vi "Find Axis Instant Velocity.vi"(6 "Sample Period":dbl, 8 "Error In":errorcluster, 10 "Desired Position":dbl, 11 "Current Position":dbl) -> (0 "Error Out":errorcluster, 2 "Axis Velocity":dbl, 3 "Current Position out":dbl)   [LabVIEW 2013]
doc: "This sub-VI determines the instantaneous velocity to send to the motors based on the axis position read\nby the encoders and the position commanded by the system."
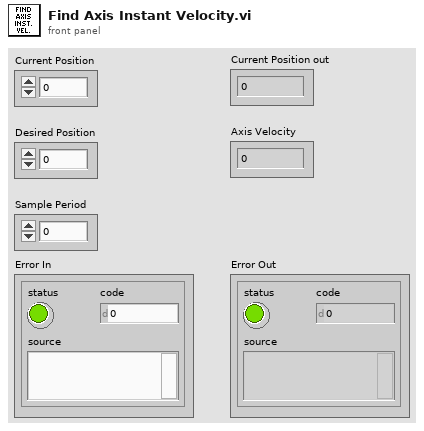
[diagram p1: front panel]
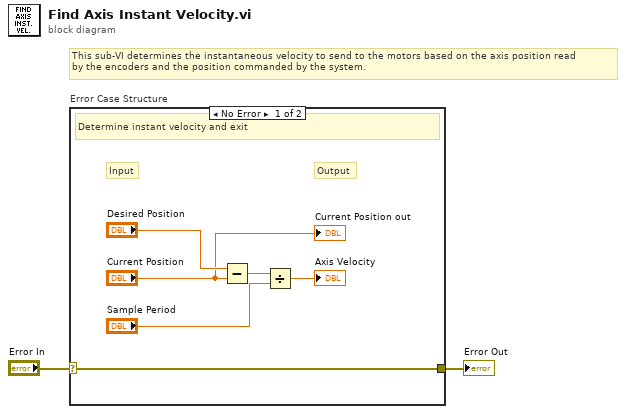
[diagram p0: block diagram]
diagram:
  # "This sub-VI determines the instantaneous velocity to send to the motors based on the axis position read\nby the encoders and the position commanded by the system."
  n1 = case "Error Case Structure" shown="No Error" "Error In" {
    selector: "Error In" -> [w8 w9]
    tunnel: [w8 w9] -> w1
    frame No Error {
      # "Output"
      # "Input"
      # "Determine instant velocity and exit"
      n2 = Subtract(x="Desired Position", y="Current Position") -> (x-y=w6:dbl)
      n3 = Divide(x=w6, y="Sample Period") -> (x/y=→"Axis Velocity":dbl)
      "Current Position out" <- "Current Position"
    }
    frame Error {
      # "Pass through and exit"
    }
  }
  "Error Out" <- w1
